vi "Bind Tab Page Controls.vi"(11 "Page in":refnum<vi>) -> (1 "Valve Control Indexes":i32[](array[numeric]), 2 "Event Registrations":refnum<event-registration>)   [LabVIEW 2015]
uses:
  Valve Name Enum.ctl
  Sensors/Sensor Enum.ctl
  Valve Button Mapping Global Action.ctl
  Sensor Indicator Map Action.ctl
panel:
  in  "Sensor Enum":T1
  in  "Valve Enum":T2
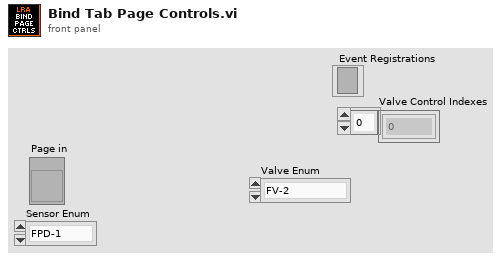
[diagram p1: front panel]
types:
  T1 = typedef "Sensor Enum.ctl" = enum16{"FPD-1", "FPD-2", "FPD-3", "OPD-1", "OPD-2", "OPD-3", "AP-1", "PC-1", "PC-2", "VBAT", "VCOMP", "ICOMP", "TC-1", "TC-COMP"}
  T2 = typedef "Valve Name Enum.ctl" = enum16{"FV-2", "FV-3", "FV-4", "OV-2", "OV-3", "OV-4", "NV-2", "COMP"}
  T3 = typedef "Sensor Indicator Map Action.ctl" = enum16{"Get", "Set"}
  T4 = typedef "Valve Button Mapping Global Action.ctl" = enum16{"Get", "Set", "Init", "Reset All", "Reset to Standby"}
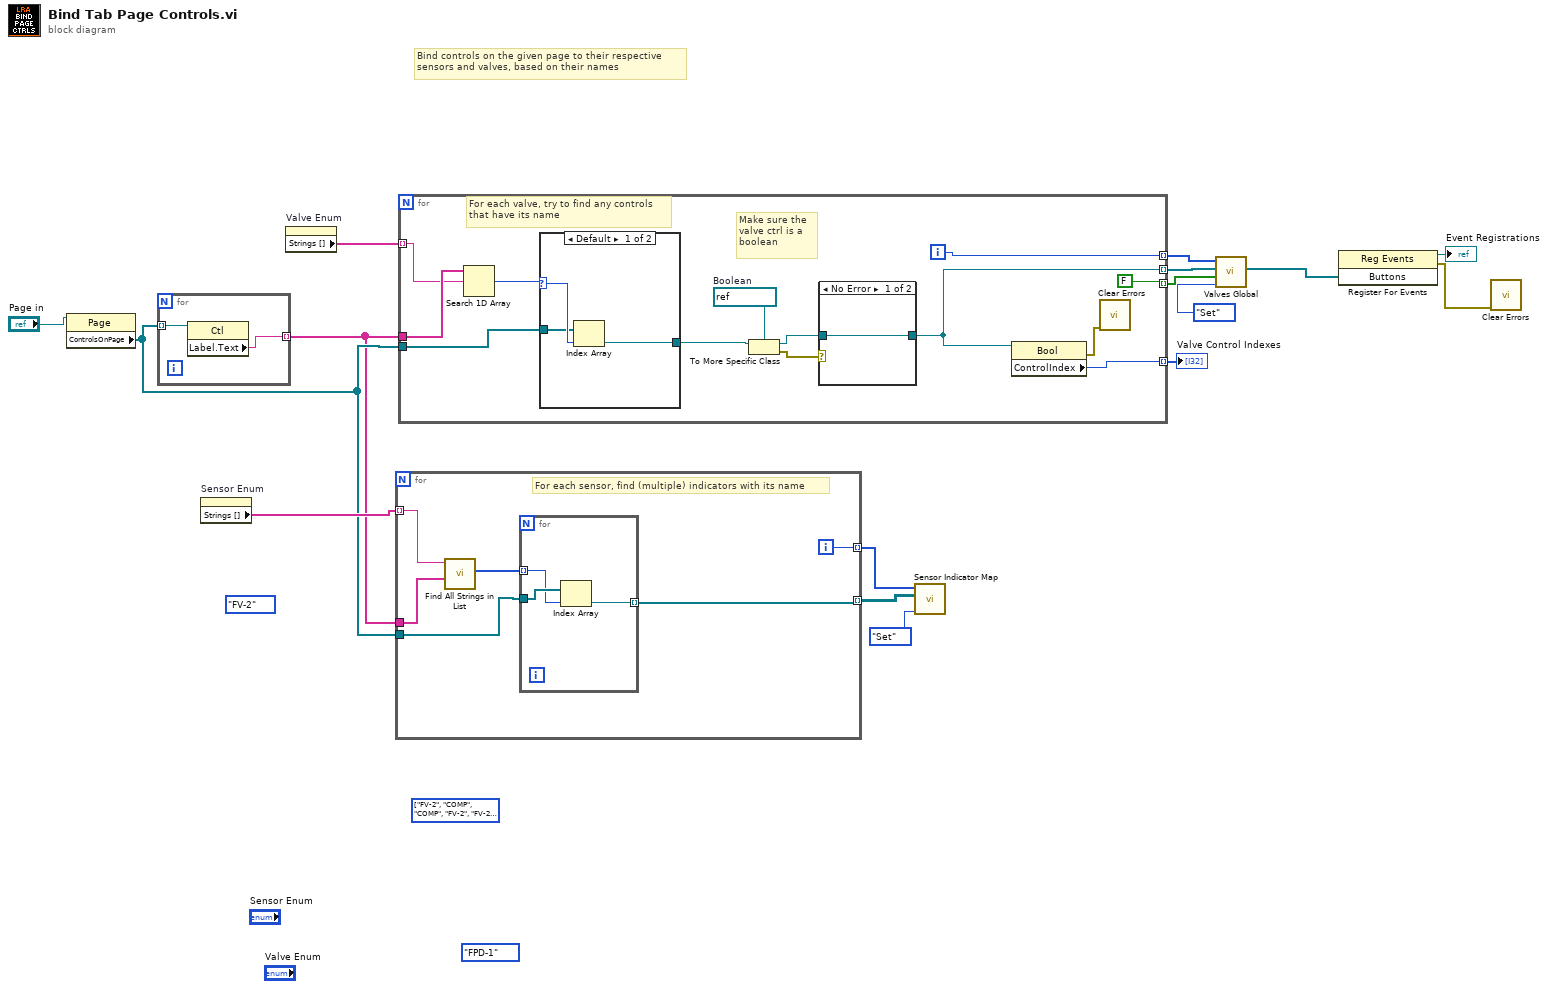
[diagram p0: block diagram]
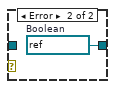
[diagram p2: hidden frame]
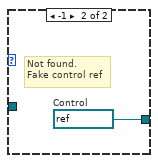
[diagram p3: hidden frame]
diagram:
  (unwired) Valve_Name_Enum."FV-2" ("Enum")
  (unwired) Sensor_Enum."FPD-1" ("Sensor Enum")
  (unwired) T2[] [enum."FV-2", enum."COMP", enum."COMP", enum."FV-2", enum."FV-2", enum."COMP", enum."COMP"] items=["FV-2", "FV-3", "FV-4", "OV-2", "OV-3", "OV-4", "NV-2", "COMP"] ("Valves")
  # "Bind controls on the given page to their respective \nsensors and valves, based on their names"
  n1 = property class="Page"(reference="Page in") -> ("ControlsOnPage"=w10:refnum<vi>[])  [unwired: 1 in, 2 out]
  n2 = for {
    tunnel: w10 -> [w18] mode=indexing
    tunnel: [w17] -> w9 mode=indexing
    n3 = property class="Ctl"(reference=w18) -> ("Label.Text"=w17:string)  [unwired: 1 in, 2 out]
  }
  n4 = property on="Sensor Enum" class="Enum (strict)"() -> ("Strings []"=w11:string[])  [unwired: 2 in, 2 out]
  n5 = property on="Valve Enum" class="Enum (strict)"() -> ("Strings []"=w15:string[])  [unwired: 2 in, 2 out]
  n6 = for {
    tunnel: w11 -> [w23] mode=indexing
    tunnel: w10 -> [w21]
    tunnel: w9 -> [w24]
    tunnel: [w20] -> w7 mode=indexing
    tunnel: [w19] -> w8 mode=indexing
    i -> [w19]
    # "For each sensor, find (multiple) indicators with its name"
    n7 = call "Find All Strings in List.vi"("List to search"=w24, "String"=w23) -> ("Matches"=w22:i32[])  [unwired: 9 in]
    n8 = for {
      tunnel: w22 -> [w26] mode=indexing
      tunnel: w21 -> [w27]
      tunnel: [w25] -> w20 mode=indexing
      n9 = Index Array(array=w27, index=w26) -> (element=w25:refnum<vi>)
    }
  }
  n10 = for {
    tunnel: w15 -> [w39] mode=indexing
    tunnel: w9 -> [w40]
    tunnel: [w38] -> w14 mode=indexing
    tunnel: [w31] -> w12 mode=indexing
    tunnel: w10 -> [w36]
    tunnel: [w30] -> w3 mode=indexing
    tunnel: [FALSE] -> w1 mode=indexing
    i -> [w38]
    w34 = refnum<vi> refnum  # Boolean
    # "Make sure the \nvalve ctrl is a \nboolean"
    # "For each valve, try to find any controls\nthat have its name"
    n11 = Search 1D Array(1D array=w40, element=w39) -> (index of element=w37:i32)  [unwired: 1 in]
    n12 = case shown="Default" w37 {
      selector: w37 -> [w45 _]
      tunnel: w36 -> [w44 _]
      tunnel: [w43 w46] -> w35
      frame Default {
        n13 = Index Array(array=w44, index=w45) -> (element=w43:refnum<vi>)
      }
      frame -1 {
        w46 = refnum<vi> refnum  # Control
        # "Not found.\nFake control ref"
      }
    }
    n14 = To More Specific Class(target class=w34, reference=w35) -> (specific class reference=w32:refnum<vi>, error out=w33:errorcluster)  [unwired: 1 in]
    n15 = case shown="No Error" w33 {
      tunnel: w32 -> [w41 _]
      tunnel: [w41 w42] -> w31
      frame No Error {
      }
      frame Error {
        w42 = refnum<vi> refnum  # Boolean
      }
    }
    n16 = property class="Bool"(reference=w31) -> (error out=w29:errorcluster, "ControlIndex"=w30:i32)  [unwired: 1 in, 1 out]
    n17 = call <vilib>:"Clear Errors.vi"("error in (no error)"=w29) -> ()  [unwired: 5 in, 2 out]
  }
  "Valve Control Indexes" <- w3
  n18 = call "Sensor Indicator Map.vi"("Action"=Sensor_Indicator_Map_Action."Set", "Control Lists In"=w7, "Sensor List In"=w8) -> ()  [unwired: 7 in, 2 out]
  n19 = call "Valves Global.vi"("Action"=Valve_Button_Mapping_Global_Action."Set", "Valve States"=w1, "Valve Buttons"=w12, "Valves"=w14) -> ("Buttons"=w5:refnum<vi>[])  [unwired: 4 in, 3 out]
  n20 = register-events(w5) -> (reference out=→"Event Registrations":refnum<event-registration>, error out=w2:errorcluster)  [unwired: 2 in]
  n21 = call <vilib>:"Clear Errors.vi"("error in (no error)"=w2) -> ()  [unwired: 5 in, 2 out]
